vi "XML Script - ControlTerm.vi"(0 "x":i32=-1, 1 "y":i32=-1, 6 "ControlName":string) -> (5 "name (wire source)":string, 7 "XML Script Command - ControlTerm":string)   [LabVIEW 2017]
uses:
  <vilib>/_script/XML Scripting/XML Script Tag.ctl
  <vilib>/_script/XML Scripting/XML Script Attribute.ctl
panel:
  # "position"
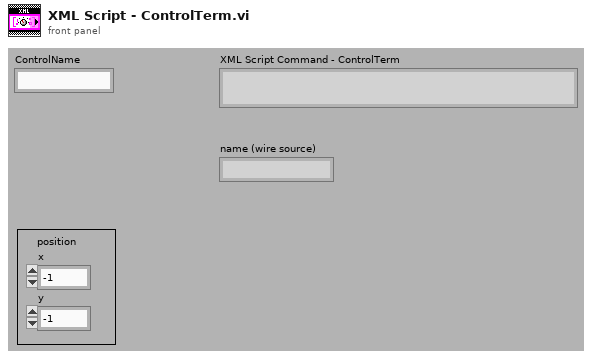
[diagram p1: front panel]
types:
  T1 = typedef "XML Script Attribute.ctl" = enum16{"name", "style", "path", "position", "in", "out", "width", "height", "index", "value", "default", "location", "offset", "typeindex", "size", "source", "destination", "indicator", "type", "controlname", "label", "conpaneidx", "mode", "description", "hasCondTerm", "linkIdentity", "caseselectortype", "concatInputs", "inName", "instantiationpath", "loopCondition", "IndexMode", "formulaInputs", "formulaOutputs", "msnFuncName", "msnIsDynamic", "msnIsODEUserFunction", "ignoreSearchDialog"}
  T2 = typedef "XML Script Tag.ctl" = enum16{"Script", "Function", "SubVI", "GrowableFunction", "Structure", "MultiframeStructure", "Frame", "Tunnel", "ShiftRegister", "Constant", "Control", "Terminal", "Wire", "StaticVIReference", "ControlTerminal", "CompoundArithmetic", "FlatSequence", "FlatSequenceFrame", "MathScriptCallByRef", "BuildArray", "GenericSubVI", "MathScriptNode"}
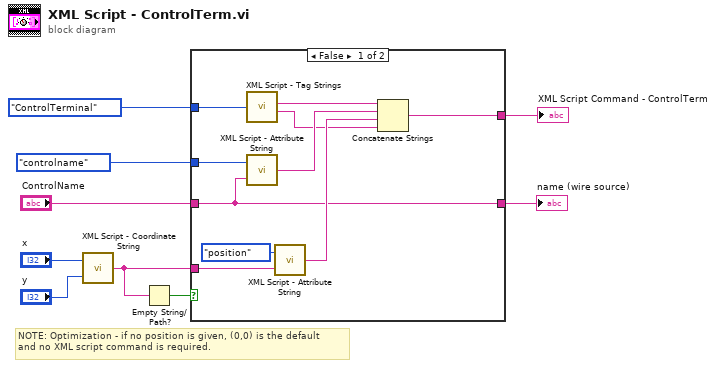
[diagram p0: block diagram]
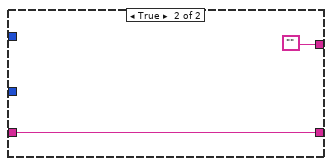
[diagram p2: hidden frame]
diagram:
  # "NOTE: Optimization - if no position is given, (0,0) is the default\nand no XML script command is required."
  n1 = call <vilib>:"XML Script - Coordinate String.vi"("y"="y", "x"="x") -> ("(x,y)"=w3:string)
  n2 = Empty String/Path?(string/path=w3) -> (empty?=w1:bool)
  n3 = case shown="False" w1 {
    tunnel: XML_Script_Tag."ControlTerminal" ("XML Script Tag") -> [w18 _]
    tunnel: XML_Script_Attribute."controlname" ("XML Script Attribute") -> [w16 _]
    tunnel: "ControlName" -> [w11 w20]
    tunnel: [w10 ""] -> w4
    tunnel: w3 -> [w12 _]
    tunnel: [w11 w20] -> w2
    frame False {
      n4 = call <vilib>:"XML Script - Tag Strings.vi"("XML Script Tag"=w18) -> ("XML String - Begin Tag"=w17:string, "XML String - End Tag"=w13:string)  [unwired: 2 in]
      n5 = call <vilib>:"XML Script - Attribute String.vi"("Attribute String"=w11, "XML Script Attribute"=w16) -> ("XML Script - Attribute String"=w15:string)
      n6 = call <vilib>:"XML Script - Attribute String.vi"("Attribute String"=w12, "XML Script Attribute"=XML_Script_Attribute."position") -> ("XML Script - Attribute String"=w14:string)
      n7 = Concatenate Strings(w17, w15, w14, w13) -> (w10:string)
    }
    frame True {
    }
  }
  "XML Script Command - ControlTerm" <- w4
  "name (wire source)" <- w2
